vi "Async Action.vi"(8 "error in (no error)":errorcluster, 9 "Message Data":variant, 10 "Message":string, 11 "Mock Async Handler Process In":refnum<class "Mock Async Handler Process.lvclass">) -> (0 "error out":errorcluster)   [LabVIEW 2020, in "Mock Async Handler Process.lvclass"]
doc: "The specific action implemented in the asynchronous action. Multiple different actions may be supported by using the Message and Message Data input to separate them. Any number of actions may run in parallell running the same or different actions. If this method throws an error, the error will be sent to the error handler configured for the process. \nCare needs to be taken so that this action is cancelled if the process is stopped. This may be detected by e.g. observing the Lifecycle: Stopped/Finished broadcast or polling the Get Lifecycle State.vi."
uses:
  Mock Async Handler Process.lvclass
  Mock Async Handler Process.lvclass/Mock Async Handler Process.ctl
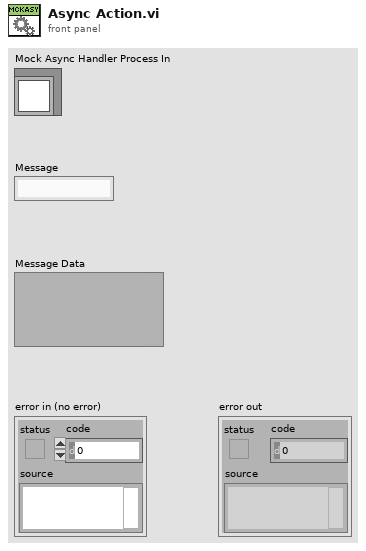
[diagram p1: front panel]
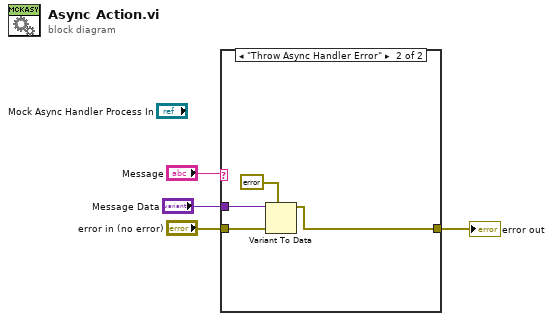
[diagram p0: block diagram]
diagram:
  n1 = case shown="\"Throw Async Handler Error\"" "Message" {
    tunnel: "error in (no error)" -> [w5 w9]
    tunnel: "Message Data" -> [_ w8]
    tunnel: [w5 w6] -> w1
    frame Default {
    }
    frame "Throw Async Handler Error" {
      n2 = Variant To Data(error in=w9, type=errorcluster {"status"=FALSE, "code"=0, "source"=""} ("error in (no error)"), Variant=w8) -> (data=w6:errorcluster)  [unwired: 1 out]
    }
  }
  "error out" <- w1
